vi "Ramp Generation.vi"() -> ()   [LabVIEW 2024]
panel:
  out "Ramp output":waveform(dbl)(graph)
  in  "Time Span":dbl
  in  "Max":dbl
  in  "# Points":dbl
  in  "Min":dbl
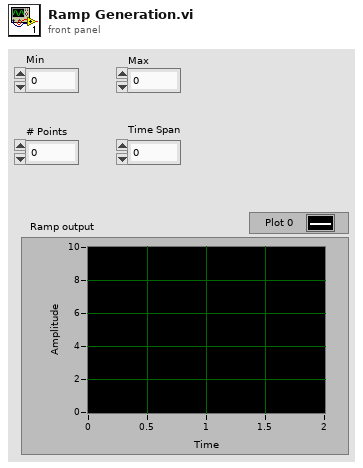
[diagram p1: front panel]
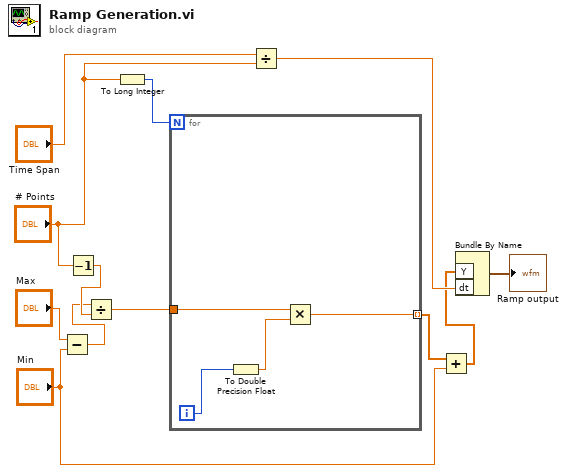
[diagram p0: block diagram]
diagram:
  n1 = Subtract(x="Max", y="Min") -> (x-y=w9:dbl)
  n2 = Decrement(x="# Points") -> (x-1=w10:dbl)
  n3 = Divide(x=w9, y=w10) -> (x/y=w8:dbl)
  n4 = To Long Integer(number="# Points") -> (32bit integer=w12:i32)
  n5 = for {
    N: w12 -> [_]
    tunnel: w8 -> [w16]
    tunnel: [w13] -> w3 mode=indexing
    i -> [w15]
    n6 = To Double Precision Float(number=w15) -> (double precision float=w14:dbl)
    n7 = Multiply(x=w16, y=w14) -> (x*y=w13:dbl)
  }
  n8 = Divide(x="Time Span", y="# Points") -> (x/y=w5:dbl)
  n9 = Add(x=w3, y="Min") -> (x+y=w1:dbl[])
  n10 = Bundle By Name("Y"=w1, "dt"=w5) -> (→"Ramp output":waveform(dbl))  [unwired: 1 in]
